vi "FTW-Endpoint-Core-SetSocketOption.vi"(0 "FTW Endpoint":refnum<class "FTW-Endpoint.lvclass">, 5 "Option Level":string, 7 "Option":string, 9 "Value":i32, 11 "error in":errorcluster) -> (4 "FTW Endpoint out":refnum<class "FTW-Endpoint.lvclass">, 15 "error out":errorcluster)   [LabVIEW 2012, in "FTW-Actor.lvlib" / "FTW-Endpoint.lvclass"]
uses:
  FTW-Endpoint.lvclass
  FTW-Endpoint.lvclass/FTW-Endpoint.ctl
panel:
  # "Inputs"
  # "Outputs"
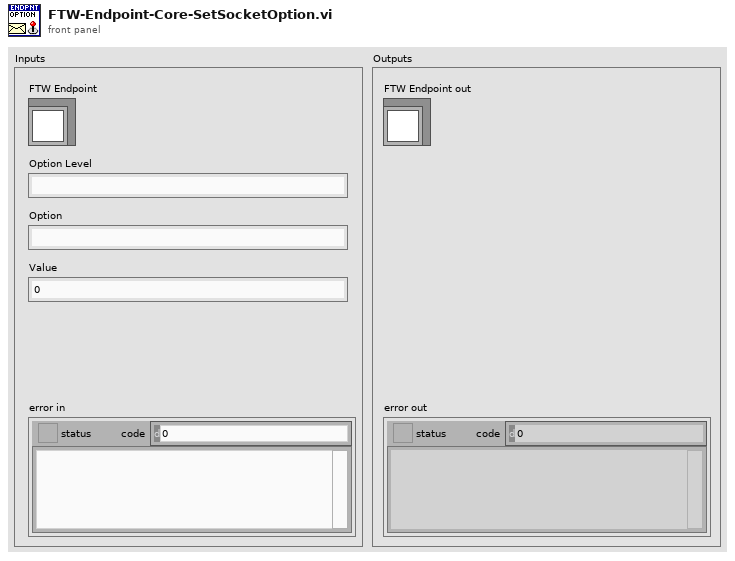
[diagram p1: front panel]
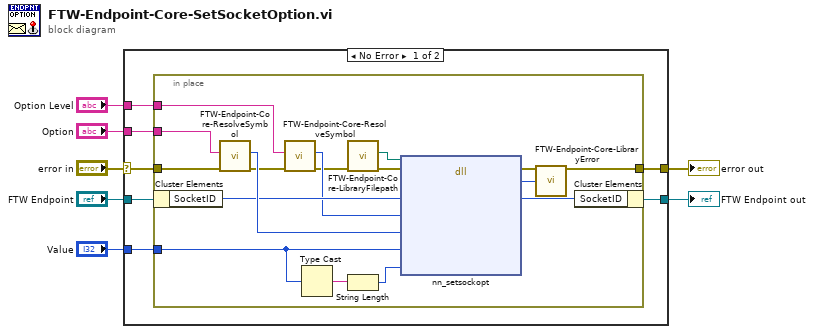
[diagram p0: block diagram]
diagram:
  n1 = case shown="No Error" "error in" {
    selector: "error in" -> [w12 w32]
    tunnel: "FTW Endpoint" -> [w14 w33]
    tunnel: [w11 w32] -> w6
    tunnel: [w13 w33] -> w5
    tunnel: "Option" -> [w10 _]
    tunnel: "Value" -> [w9 _]
    tunnel: "Option Level" -> [w8 _]
    frame No Error {
      n2 = in-place {
        in-place-border: w12 -> [w16]
        in-place-border: [w23] -> w11
        in-place-border: w10 -> [w21]
        in-place-border: w9 -> [w20]
        in-place-border: w8 -> [w15]
        n3 = in-place-cluster #1(w14) -> ("SocketID"=w25:i64)
        n4 = call "FTW-Endpoint-Core-ResolveSymbol.vi"("error in"=w16, "Symbol"=w21) -> ("error out"=w17:errorcluster, "Symbol Value"=w29:i32)  [unwired: 8 in]
        n5 = call "FTW-Endpoint-Core-ResolveSymbol.vi"("error in"=w17, "Symbol"=w15) -> ("error out"=w19:errorcluster, "Symbol Value"=w22:i32)  [unwired: 8 in]
        n6 = Type Cast(x=w20) -> (*(type *) &x=w28:string)  [unwired: 1 in]
        n7 = call "FTW-Endpoint-Core-LibraryFilepath.vi"("error in"=w19) -> ("error out"=w18:errorcluster, "Library Filepath"=w26:path)  [unwired: 8 in, 1 out]
        n8 = String Length(string=w28) -> (length=w27:i32)
        n9 = dll-call lib="?" fn="nn_setsockopt"(path in=w26, error in=w18, "SocketID"=w25, "Option Level"=w22, "Option"=w29, "Option Value"=w20, "Option Value Length"=w27) -> (error out=w30:errorcluster, "Return Value"=w31:i64, "SocketID"=w24:i64)  [unwired: 5 in, 1 out]
        n10 = call "FTW-Endpoint-Core-LibraryError.vi"("error in"=w30, "Return Value"=w31) -> ("error out"=w23:errorcluster)  [unwired: 13 in]
        n11 = in-place-cluster #1("SocketID"=w24) -> (w13:refnum<class "FTW-Endpoint.lvclass">)
      }
    }
    frame Error {
    }
  }
  "error out" <- w6
  "FTW Endpoint out" <- w5
